vi "Solve1.vi"(8 "Error In":errorcluster, 11 "object in":refnum<class "2024_1.lvclass">) -> (0 "Error Out":errorcluster, 2 "Result":u64, 3 "object out":refnum<class "2024_1.lvclass">)   [LabVIEW 2023, in "2024_1.lvclass"]
uses:
  2024_1.lvclass
  2024_1.lvclass/2024_1.ctl
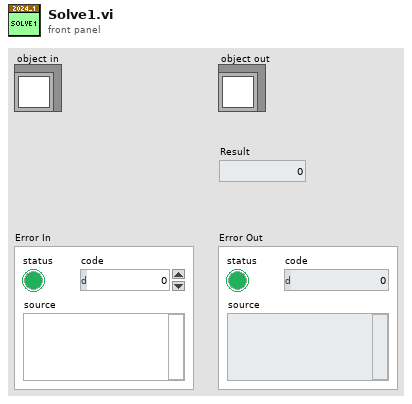
[diagram p1: front panel]
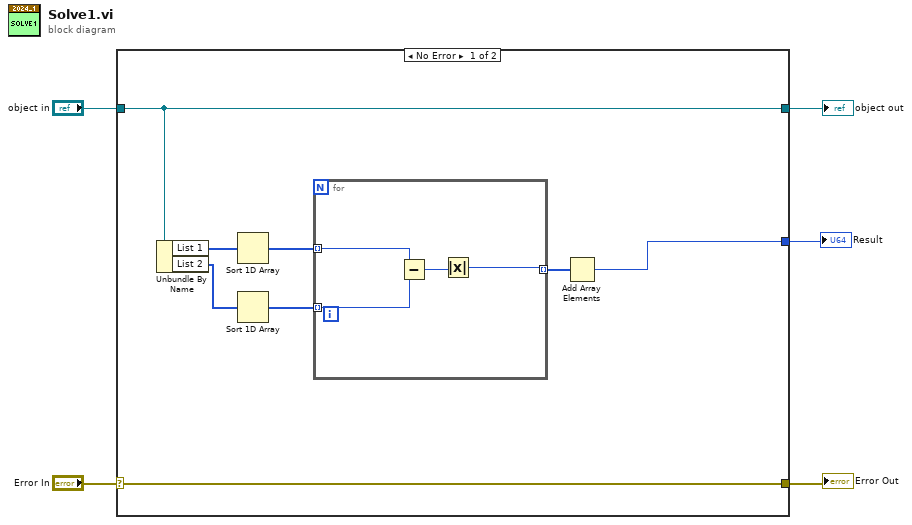
[diagram p0: block diagram]
diagram:
  n1 = case shown="No Error" "Error In" {
    selector: "Error In" -> [w13 w19]
    tunnel: [w13 w19] -> w4
    tunnel: [w12 w18] -> w2
    tunnel: "object in" -> [w12 w18]
    tunnel: [w6 _] -> w1
    frame No Error {
      n2 = Unbundle By Name(w12) -> ("List 1"=w11:i64[], "List 2"=w9:i64[])
      n3 = Sort 1D Array(array=w11) -> (sorted array=w10:i64[])
      n4 = Sort 1D Array(array=w9) -> (sorted array=w8:i64[])
      n5 = for {
        tunnel: w10 -> [w17] mode=indexing
        tunnel: w8 -> [w16] mode=indexing
        tunnel: [w14] -> w7 mode=indexing
        n6 = Subtract(x=w17, y=w16) -> (x-y=w15:i64)
        n7 = Absolute Value(x=w15) -> (abs(x)=w14:i64)
      }
      n8 = Add Array Elements(numeric array=w7) -> (sum=w6:i64)
    }
    frame Error {
    }
  }
  "Error Out" <- w4
  "object out" <- w2
  "Result" <- w1
